vi "status in device case.vi"(0 "Data cluster in":T1, 5 "current case":string, 7 "Arguments":string, 9 "raw saving path":string, 11 "shot number":i32, 12 "add variables to subscribe":string) -> (3 "NOT in scan mode?":bool, 4 "Data cluster out":T1, 6 "Device State":string, 10 "NOT a new shot":bool, 15 "remote subscriber string":string)   [LabVIEW 2009]
uses:
  dataCluster.ctl
  <vilib>/vision/Image Controls.llb/IMAQ Image.ctl
  DataQueueTypeDef.ctl
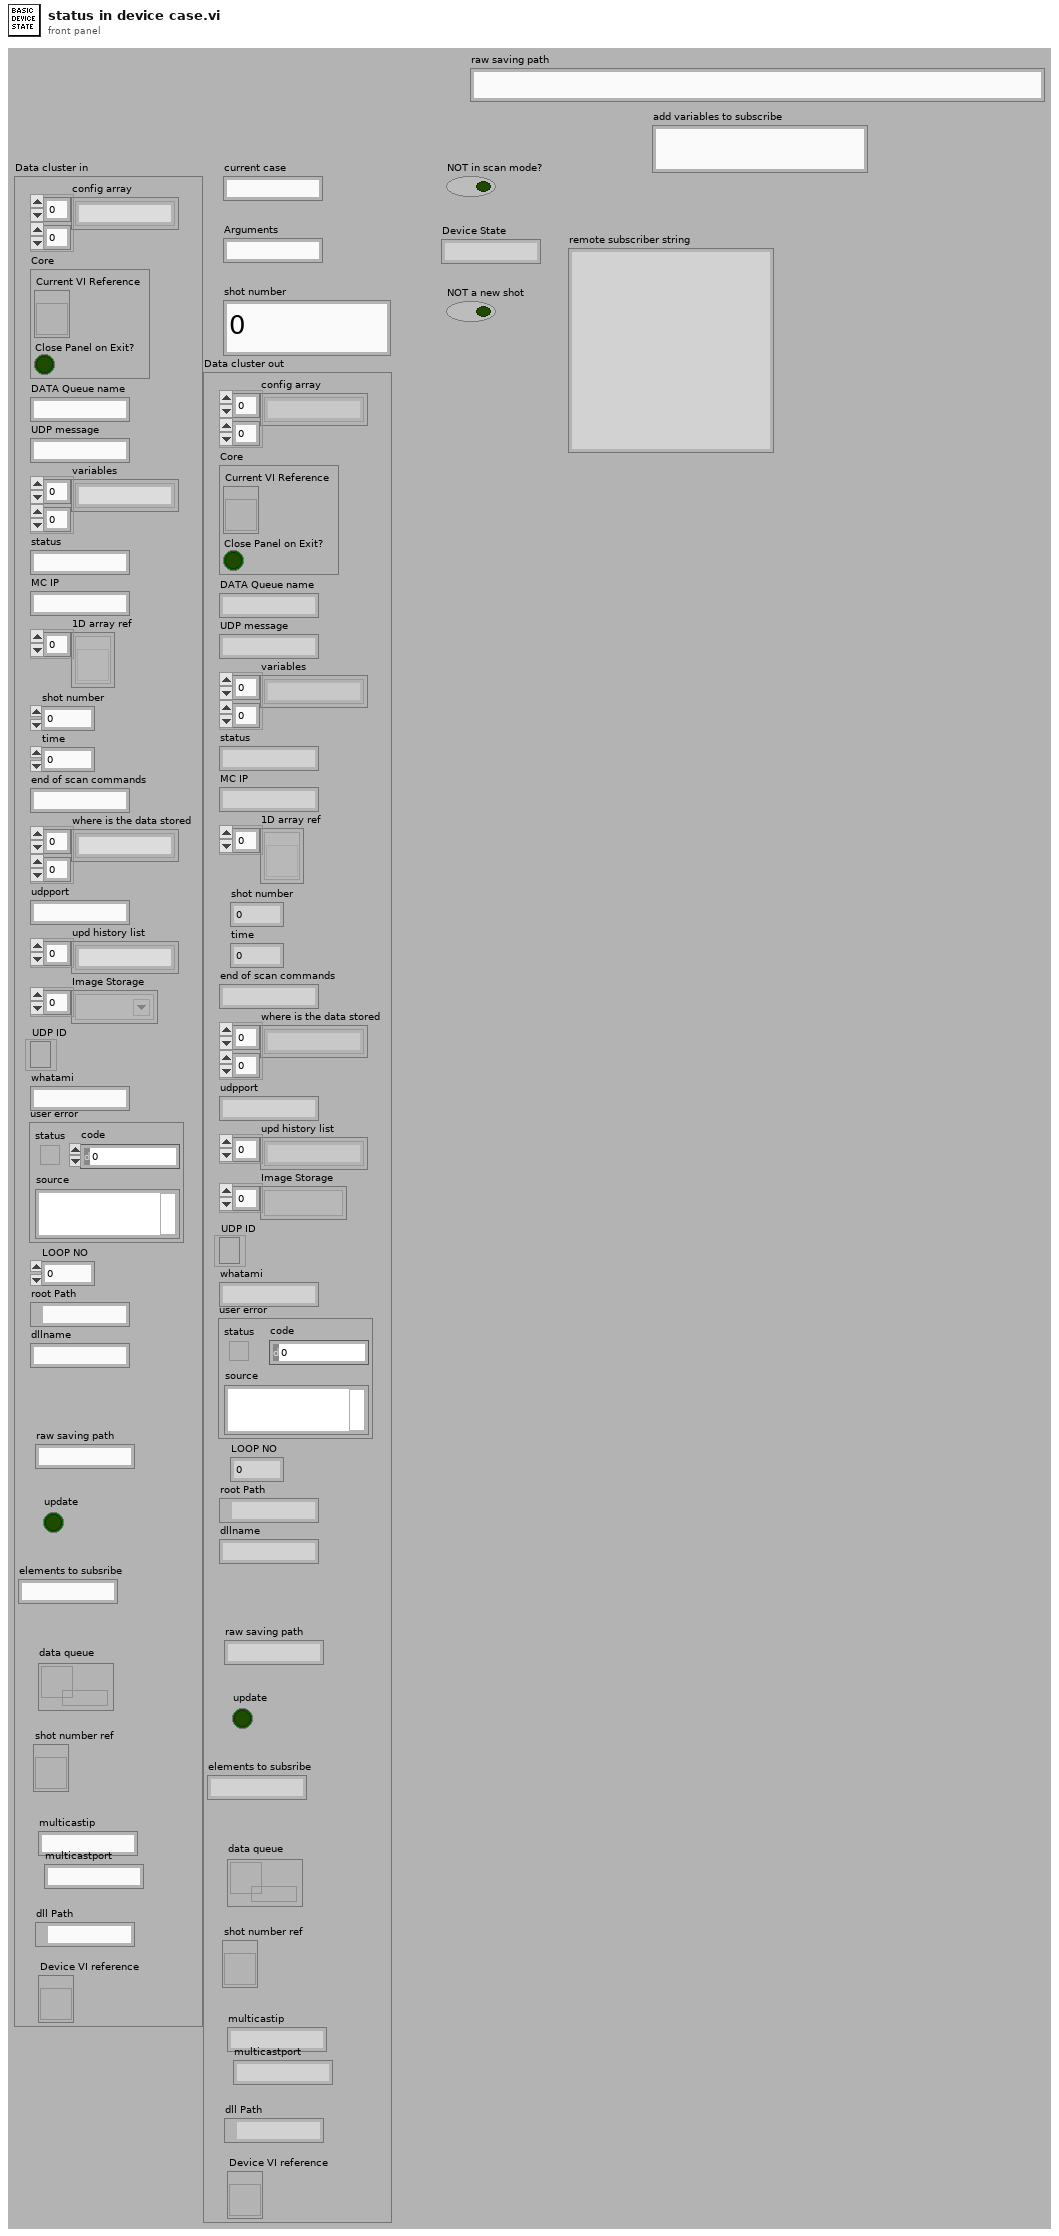
[diagram p1: front panel]
types:
  T1 = typedef "dataCluster.ctl" = cluster{"config array":string[][], "Core":cluster{"Current VI Reference":refnum<vi>, "Close Panel on Exit?":bool}, "DATA Queue name":string, "UDP message":string, "variables":string[][], "status":string, "MC IP":string, "1D array ref":refnum<vi>[], "shot number":i32, "time":u32, "end of scan commands":string, "where is the data stored":string[][], "udpport":string, "upd history list":string[], "Image Storage":T2[], "UDP ID":refnum<k16>, "whatami":string, "user error":errorcluster, "LOOP NO":u32, "root Path":path, "dllname":string, "raw saving path":string, "update":bool, "elements to subsribe":string, "data queue":refnum<queue>, "shot number ref":refnum<vi>, "multicastip":string, "multicastport":string, "dll Path":path, "Device VI reference":refnum<vi>}
  T2 = typedef "IMAQ Image.ctl" = refnum<image>
  T3 = typedef "DataQueueTypeDef.ctl" = cluster{"connection ID":refnum<k5>, "remote address":string, "Subscriber list":string[], "wait":bool, "port":u16}
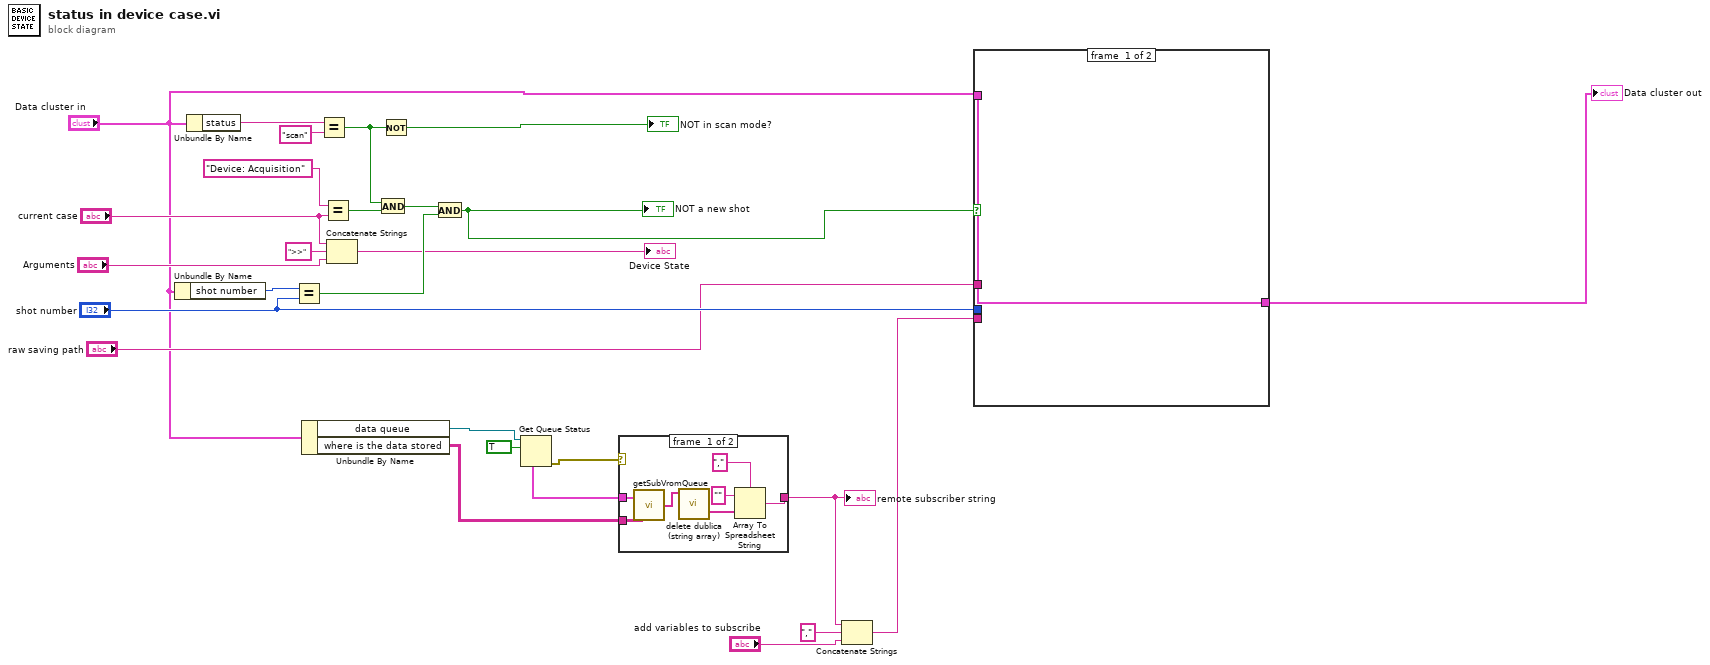
[diagram p0: block diagram]
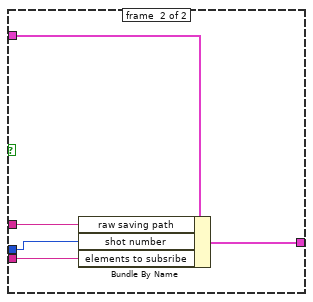
[diagram p2: hidden frame]
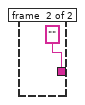
[diagram p3: hidden frame]
diagram:
  n1 = Unbundle By Name("Data cluster in") -> ("shot number"=w22:i32)
  n2 = Unbundle By Name("Data cluster in") -> ("status"=w18:string)
  n3 = Equal?(x=w22, y="shot number") -> (x = y?=w26:bool)
  n4 = Unbundle By Name("Data cluster in") -> ("data queue"=w7:refnum<queue>, "where is the data stored"=w9:string[][])
  n5 = Equal?(x=w18, y="scan") -> (x = y?=w24:bool)
  n6 = Equal?(x="Device: Acquisition" ("y"), y="current case") -> (x = y?=w27:bool)
  n7 = Concatenate Strings("current case", ">>" ("string"), "Arguments") -> (→"Device State":string)
  n8 = And(x=w24, y=w27) -> (x .and. y?=w25:bool)
  n9 = Not(x=w24) -> (.not. x?=→"NOT in scan mode?":bool)
  n10 = And(x=w25, y=w26) -> (x .and. y?=w5:bool)
  "NOT a new shot" <- w5
  n11 = Get Queue Status(queue=w7, return elements? (F)=TRUE) -> (error out=w8:errorcluster, elements=w10:T3[])  [unwired: 1 in, 6 out]
  n12 = case shown="No Error" w8 {
    tunnel: w10 -> [w33 _]
    tunnel: [w29 "" ("spreadsheet string")] -> w14
    tunnel: w9 -> [w28 _]
    frame #0 {
      n13 = call "getSubVromQueue.vi"("where is the data stored"=w28, "elements"=w33) -> ("Array"=w34:string[])
      n14 = call "delete dublica (string array).vi"("Array in"=w34) -> ("Array out"=w32:string[])  [unwired: 10 in]
      n15 = Array To Spreadsheet String(delimiter (Tab)=",", array=w32, 3:"" ("format string")) -> (spreadsheet string=w29:string)
    }
    frame #1 {
    }
  }
  "remote subscriber string" <- w14
  n16 = Concatenate Strings(w14, "," ("string"), "add variables to subscribe") -> (w6:string)
  n17 = case shown="True" w5 {
    tunnel: w6 -> [_ w41]
    tunnel: "shot number" -> [_ w40]
    tunnel: "raw saving path" -> [_ w39]
    tunnel: "Data cluster in" -> [w36 w38]
    tunnel: [w36 w37] -> w1
    frame #0 {
    }
    frame #1 {
      n18 = Bundle By Name(cluster=w38, "raw saving path"=w39, "shot number"=w40, "elements to subsribe"=w41) -> (w37:T1)
    }
  }
  "Data cluster out" <- w1
